vi "Version to String.vi"(4 "Version":T1, 5 "Pre-Release (None)":string) -> (7 "Version String":string)   [LabVIEW 2020, in "Builder Core.lvlib"]
uses:
  Builder Core.lvlib
  Version.ctl
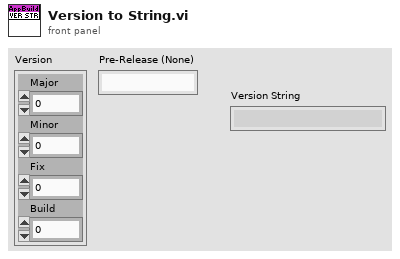
[diagram p1: front panel]
types:
  T1 = typedef "Builder Core.lvlib/Version.ctl" = cluster{"Major":u16, "Minor":u16, "Fix":u16, "Build":u16}
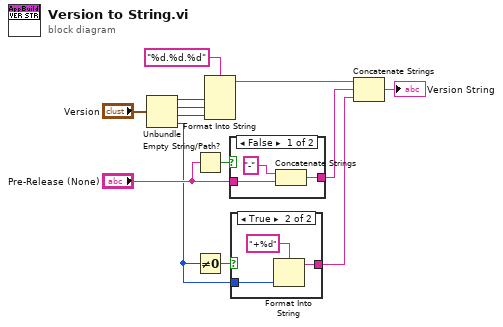
[diagram p0: block diagram]
diagram:
  n1 = Unbundle("Version") -> ("Major"=w12:u16, "Minor"=w11:u16, "Fix"=w10:u16, "Build"=w5:u16)
  n2 = Empty String/Path?(string/path="Pre-Release (None)") -> (empty?=w8:bool)
  n3 = Not Equal To 0?(x=w5) -> (x != 0?=w6:bool)
  n4 = Format Into String(format string="%d.%d.%d", w12, w11, w10) -> (resulting string=w4:string)  [unwired: 2 in, 1 out]
  n5 = case shown="False" w8 {
    tunnel: "Pre-Release (None)" -> [w16 _]
    tunnel: [w14 _] -> w3
    frame False {
      n6 = Concatenate Strings("-" ("string"), w16) -> (w14:string)
    }
    frame True {
    }
  }
  n7 = case shown="True" w6 {
    tunnel: w5 -> [_ w18]
    tunnel: [_ w17] -> w2
    frame False {
    }
    frame True {
      n8 = Format Into String(format string="+%d", w18) -> (resulting string=w17:string)  [unwired: 2 in, 1 out]
    }
  }
  n9 = Concatenate Strings(w4, w3, w2) -> (→"Version String":string)
